vi "Write Tau to U.vi"(7 "State":enum16{"Write", "Close"}(ring), 9 "Time":timestamp, 10 "taus":sgl[](array[numeric])) -> (0 "error out":errorcluster)   [LabVIEW 2011]
uses:
  File IO/File Utilities.lvlib
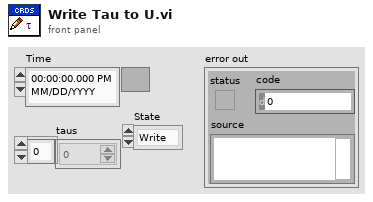
[diagram p1: front panel]
types:
  T1 = enum16{"open", "replace", "create", "open or create", "replace or create", "replace or create with confirmation"}
  T2 = enum16{"big-endian, network order", "native, host order", "little-endian"}
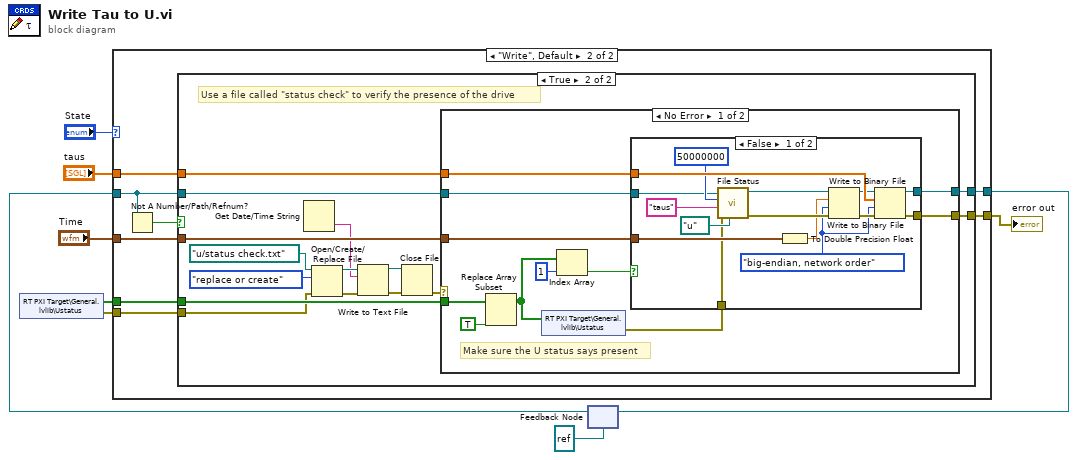
[diagram p0: block diagram]
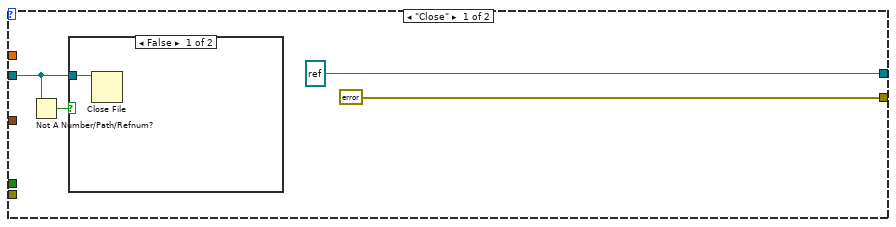
[diagram p2: hidden frame]
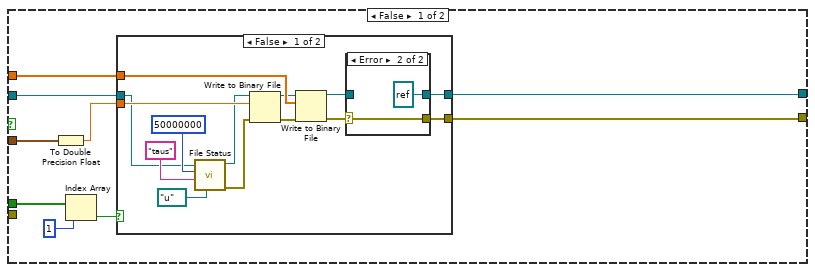
[diagram p4: hidden frame]
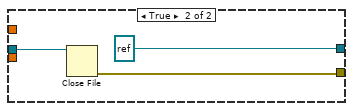
[diagram p6: hidden frame]
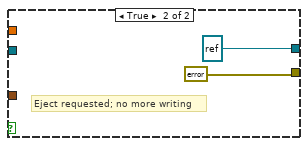
[diagram p7: hidden frame]
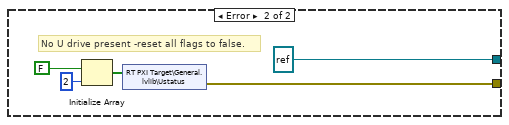
[diagram p8: hidden frame]
diagram:
  n1 = shared-variable "RT PXI Target\\General.lvlib\\Ustatus"() -> (w8:bool[], error out=w1:errorcluster)  [unwired: 1 in]
  n2 = feedback #1(refnum<file> refnum ("refnum out")) -> (w7:refnum<file>)
  n3 = case shown="\"Write\", Default" "State" {
    tunnel: w7 -> [w13 w22]
    tunnel: [refnum<file> refnum ("refnum out") w20] -> w5
    tunnel: "Time" -> [_ w19]
    tunnel: "taus" -> [_ w18]
    tunnel: w8 -> [_ w17]
    tunnel: [errorcluster {"status"=FALSE, "code"=0, "source"=""} ("error out") w16] -> w2
    tunnel: w1 -> [_ w15]
    frame "Close" {
      n4 = Not A Number/Path/Refnum?(number/path/refnum=w13) -> (NaN/Path/Refnum?=w12:bool)
      n5 = case shown="False" w12 {
        tunnel: w13 -> [w14 _]
        frame False {
          n6 = Close File(refnum=w14) -> ()  [unwired: 1 in, 2 out]
        }
        frame True {
        }
      }
    }
    frame "Write", Default {
      n7 = Not A Number/Path/Refnum?(number/path/refnum=w22) -> (NaN/Path/Refnum?=w21:bool)
      n8 = case shown="True" w21 {
        tunnel: w18 -> [w28 w66]
        tunnel: w19 -> [w29 w65]
        tunnel: [w27 w67] -> w20
        tunnel: w22 -> [w31 w55]
        tunnel: w17 -> [w26 w56]
        tunnel: [w23 w54] -> w16
        tunnel: w15 -> [_ w53]
        frame False {
          n9 = To Double Precision Float(number=w29) -> (double precision float=w30:dbl)
          n10 = Index Array(array=w26, index=1) -> (element=w24:bool)
          n11 = case shown="False" w24 {
            tunnel: w31 -> [w35 w52]
            tunnel: w30 -> [w44 _]
            tunnel: w28 -> [w43 _]
            tunnel: [w39 refnum<file> refnum ("refnum out")] -> w27
            tunnel: [w32 w50] -> w23
            frame False {
              n12 = call "File Status.vi"("Data Path"=path "u:/" ("file path (use dialog)"), "prefix"="taus", "fSize"=i64 50000000, "fileRefIn"=w35) -> ("error out"=w33:errorcluster, "fileRefOut"=w34:refnum<file>)  [unwired: 6 in]
              n13 = Write to Binary File(file (use dialog)=w34, data=w44, error in=w33) -> (refnum out=w42:refnum<file>, error out=w45:errorcluster)  [unwired: 3 in, 1 out]
              n14 = Write to Binary File(file (use dialog)=w42, data=w43, error in=w45) -> (refnum out=w40:refnum<file>, error out=w41:errorcluster)  [unwired: 3 in, 1 out]
              n15 = case shown="Error" w41 {
                selector: w41 -> [w46 w48]
                tunnel: [w47 refnum<file> refnum ("refnum out")] -> w39
                tunnel: w40 -> [w47 _]
                tunnel: [w46 w48] -> w32
                frame No Error {
                }
                frame Error {
                }
              }
            }
            frame True {
              n16 = Close File(refnum=w52) -> (error out=w50:errorcluster)  [unwired: 1 in, 1 out]
            }
          }
        }
        frame True {
          # "Use a file called \"status check\" to verify the presence of the drive"
          n17 = Get Date/Time String() -> (time string=w60:string)  [unwired: 3 in, 1 out]
          n18 = Open/Create/Replace File(file path (use dialog)=path "u:/status check.txt", error in=w53, operation (0:open)=T1."replace or create") -> (refnum out=w61:refnum<file>, error out=w62:errorcluster)  [unwired: 3 in, 1 out]
          n19 = Write to Text File(file (use dialog)=w61, text=w60, error in=w62) -> (refnum out=w58:refnum<file>, error out=w59:errorcluster)  [unwired: 1 in, 1 out]
          n20 = Close File(refnum=w58, error in=w59) -> (error out=w57:errorcluster)  [unwired: 1 out]
          n21 = case shown="No Error" w57 {
            tunnel: [w78 refnum<file> refnum ("refnum out")] -> w67
            tunnel: w66 -> [w77 _]
            tunnel: w65 -> [w76 _]
            tunnel: w56 -> [w75 _]
            tunnel: w55 -> [w70 _]
            tunnel: [w69 w96] -> w54
            frame No Error {
              # "Make sure the U status says present"
              n22 = Replace Array Subset(array=w75, new element=TRUE) -> (w73:bool[])  [unwired: 1 in]
              n23 = shared-variable "RT PXI Target\\General.lvlib\\Ustatus"(w73) -> (error out=w68:errorcluster)  [unwired: 1 in]
              n24 = Index Array(array=w73, index=1) -> (element=w71:bool)
              n25 = case shown="False" w71 {
                tunnel: [w93 refnum<file> refnum ("refnum out")] -> w78
                tunnel: w77 -> [w92 _]
                tunnel: w76 -> [w91 _]
                tunnel: w70 -> [w81 _]
                tunnel: [w80 errorcluster {"status"=FALSE, "code"=0, "source"=""} ("error out")] -> w69
                tunnel: w68 -> [w79 _]
                frame False {
                  w83 = T2."big-endian, network order" ("byte order (0:big-endian, network order)")
                  n26 = call "File Status.vi"("Data Path"=path "u:/" ("file path (use dialog)"), "erriorIn"=w79, "prefix"="taus", "fSize"=i64 50000000, "fileRefIn"=w81) -> ("error out"=w88:errorcluster, "fileRefOut"=w90:refnum<file>)  [unwired: 5 in]
                  n27 = To Double Precision Float(number=w91) -> (double precision float=w84:dbl)
                  n28 = Write to Binary File(file (use dialog)=w90, data=w84, error in=w88, 9:w83) -> (refnum out=w85:refnum<file>, error out=w86:errorcluster)  [unwired: 2 in, 1 out]
                  n29 = Write to Binary File(file (use dialog)=w85, data=w92, error in=w86, 9:w83) -> (refnum out=w93:refnum<file>, error out=w80:errorcluster)  [unwired: 2 in, 1 out]
                }
                frame True {
                  # "Eject requested; no more writing"
                }
              }
            }
            frame Error {
              # "No U drive present -reset all flags to false."
              n30 = Initialize Array(FALSE, 2 ("dimension size")) -> (w97:bool[])
              n31 = shared-variable "RT PXI Target\\General.lvlib\\Ustatus"(w97) -> (error out=w96:errorcluster)  [unwired: 1 in]
            }
          }
        }
      }
    }
  }
  "error out" <- w2
  n32 = feedback-in #1(w5) -> ()
